vi "Rio_XY_Initalise_(DONE).vi"(6 "Time Passed":u32, 8 "Error In":errorcluster) -> (0 "Error Out":errorcluster, 7 "Axis Initalised":bool=TRUE)   [LabVIEW 2017]
doc: "This VI initalises the 0 values of the encoders for the X & Y axis by driving the motors into the negative limit switches.\n\nWritten by Stefan Clarkson, Robin Moore & Thomas Quinn 22/03/18."
uses:
  <vilib>/myRIO/Common/Instrument Driver Framework/myRIO v1.0/Encoder/typedefs/Encoder Signal Mode.ctl
  <vilib>/myRIO/Instrument Drivers/Onboard IO/Encoder/typedefs/Encoder Reference.ctl
  <vilib>/myRIO/Common/Instrument Driver Framework/Utilities/typedefs/myRIO Generic Hardware Reference.ctl
  <vilib>/myRIO/Common/Instrument Driver Framework/Utilities/typedefs/Hardware Version Enum.ctl
  <vilib>/myRIO/Common/Instrument Driver Framework/Utilities/typedefs/myRIO v1.0 Reference.ctl
  <vilib>/myRIO/Common/Instrument Driver Framework/Utilities/typedefs/Generic FPGA Reference.ctl
  <vilib>/myRIO/Common/Instrument Driver Framework/myRIO v1.0/Encoder/typedefs/Encoder Channels Enum.ctl
  <vilib>/myRIO/Common/Instrument Driver Framework/myRIO v1.0/Encoder/typedefs/Encoder Configuration v1.0.ctl
  <vilib>/userdefined/High Color/nirio_resource_hc.ctl
  <vilib>/myRIO/Common/Instrument Driver Framework/Utilities/vis/Is FPGA Ref Available.vi
  <vilib>/myRIO/Common/Instrument Driver Framework/myRIO v1.0/Encoder/vis/myRIO v1.1 Open Encoder.vi
  <vilib>/myRIO/Instrument Drivers/Onboard IO/Encoder/vis/Read.vi
  <vilib>/myRIO/Common/Instrument Driver Framework/Utilities/vis/Validate Channels.vi
  <vilib>/myRIO/Common/Instrument Driver Framework/myRIO v1.0/Encoder/vis/myRIO v1.0 Reserve Encoder.vi
  <vilib>/myRIO/Common/Instrument Driver Framework/myRIO v1.0/Encoder/vis/myRIO v1.0 Build MUX Configuration Encoder.vi
  <vilib>/myRIO/Common/Instrument Driver Framework/myRIO v1.0/Resource Manager/vis/myRIO v1.0 Reserve Channel List.vi
  <vilib>/myRIO/Common/Instrument Driver Framework/myRIO v1.0/Resource Manager/vis/myRIO v1.0 Create Configuration List.vi
  <vilib>/myRIO/Common/Instrument Driver Framework/myRIO v1.0/Resource Manager/vis/myRIO v1.0 Reserve Channel.vi
  <vilib>/myRIO/Common/Instrument Driver Framework/myRIO v1.0/Resource Manager/vis/myRIO v1.0 Unreserve Channel.vi
  <vilib>/myRIO/Common/Instrument Driver Framework/myRIO v1.0/Resource Manager/vis/myRIO v1.0 Build Mutex Name.vi
  <vilib>/Utility/VariantDataType/GetNumericInfo.vi
  <vilib>/Utility/error.llb/Error Cluster From Error Code.vi
  <vilib>/myRIO/Common/Instrument Driver Framework/myRIO v1.0/myRIO v1.1 Open.vi
  <vilib>/myRIO/Common/Instrument Driver Framework/Utilities/vis/IO Manager.vi
  <vilib>/myRIO/Common/Instrument Driver Framework/Utilities/vis/Configuration Manager.vi
  <vilib>/myRIO/Common/Instrument Driver Framework/myRIO v1.0/Resource Manager/vis/myRIO v1.0 Configure IO.vi
  <vilib>/myRIO/Common/Instrument Driver Framework/myRIO v1.0/myRIO v1.0 Close.vi
  <vilib>/myRIO/Common/Instrument Driver Framework/myRIO v1.0/Encoder/vis/myRIO v1.0 Configure Encoder.vi
  <vilib>/myRIO/Common/Instrument Driver Framework/myRIO v1.0/Encoder/vis/myRIO v1.0 Read Encoder.vi
  <vilib>/myRIO/Express VI/Onboard IO/Encoder/Encoder Express VI.xnode
  <vilib>/myRIO/Instrument Drivers/Onboard IO/Encoder/vis/myRIO Encoder Open.xnode
  <vilib>/myRIO/Common/Instrument Driver Framework/myRIO v1.0/Encoder/typedefs/Encoder Count Direction Enum.ctl
  <vilib>/myRIO/Instrument Drivers/Onboard IO/Encoder/Encoder.lvlib
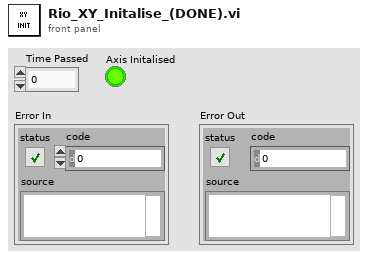
[diagram p1: front panel]
types:
  T1 = typedef "Encoder.lvlib/Encoder Reference.ctl" = cluster{"myRIO Reference":T2, "Encoder Channels Enum":T6}
  T2 = typedef "myRIO Generic Hardware Reference.ctl" = cluster{"myRIO Model":T3, "myRIO Hardware Reference":T4}
  T3 = typedef "Hardware Version Enum.ctl" = enum16{"Unknown", "myRIO-1900", "myRIO-1950", "roboRIO", "NI ELVIS RIO CM"}
  T4 = typedef "myRIO v1.0 Reference.ctl" = cluster{"Generic FPGA Reference":T5, "Allow multiple opens":bool}
  T5 = typedef "Generic FPGA Reference.ctl" = refnum<k20>
  T6 = typedef "Encoder Channels Enum.ctl" = enum16{"Not Connected", "C/ENC0", "C/ENC1", "A/ENC", "B/ENC", "DIO/ENC0", "DIO/ENC1", "DIO/ENC2", "DIO/ENC3", "DIO/ENC4"}
  T7 = typedef "Encoder Signal Mode.ctl" = enum16{"Quadrature phase signal", "Step and direction signal"}
  T8 = typedef "nirio_resource_hc.ctl" = tag
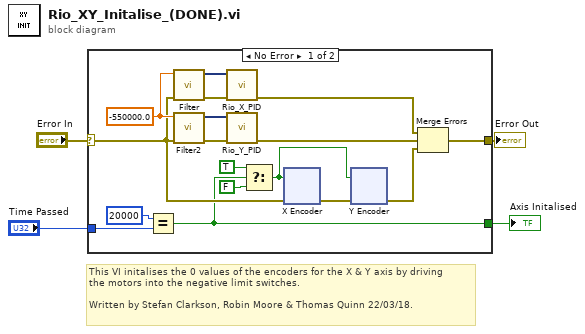
[diagram p0: block diagram]
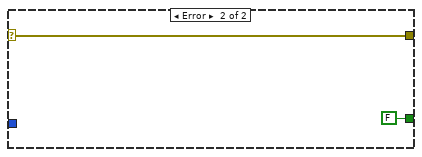
[diagram p2: hidden frame]
diagram:
  # "This VI initalises the 0 values of the encoders for the X & Y axis by driving \nthe motors into the negative limit switches.\n\nWritten by Stefan Clarkson, Robin Moore & Thomas Quinn 22/03/18."
  n1 = case shown="No Error" "Error In" {
    selector: "Error In" -> [w7 w115]
    tunnel: "Time Passed" -> [w18 _]
    tunnel: [w11 w115] -> w3
    tunnel: [w5 FALSE] -> w1
    frame No Error {
      w16 = -550000.0 ("Signal")
      n2 = Equal?(x=20000, y=w18) -> (x = y?=w5:bool)
      n3 = call "Filter"("error in (no error)"=w7, "Signal"=w16) -> ("error out"=w20:errorcluster, "Filtered Signal"=w21:dynamicdata)  [unwired: 8 in]
      n4 = call "Filter2"("error in (no error)"=w7, "Signal"=w16) -> ("error out"=w14:errorcluster, "Filtered Signal"=w15:dynamicdata)  [unwired: 8 in]
      n5 = call "Rio_X_PID.vi"("Error In"=w20, "Setpoint"=w21) -> ("Error Out"=w13:errorcluster)  [unwired: 6 in, 3 out]
      n6 = call "Rio_Y_PID.vi"("Error In"=w14, "Setpoint"=w15) -> ("Error Out"=w12:errorcluster)  [unwired: 6 in, 3 out]
      n7 = Select(t=TRUE ("Reset Counter"), s=w5, f=FALSE ("Reset Counter")) -> (s? t:f=w10:bool)
      n8 = xnode "X Encoder"("error in (no error)"=w7, "Reset Counter"=w10) -> ("error out"=w9:errorcluster)  [unwired: 3 out]
      n9 = xnode "Y Encoder"("error in (no error)"=w9, "Reset Counter"=w10) -> ("error out"=w8:errorcluster)  [unwired: 3 out]
      n10 = Merge Errors(w13, w12, w8) -> (w11:errorcluster)
    }
    frame Error {
    }
  }
  "Error Out" <- w3
  "Axis Initalised" <- w1
